vi "TIFF Add Image (array).vi"(8 "error in (no error)":errorcluster, 10 "IFD":refnum<class "IFD.lvclass">[](array[class]), 11 "TIFF in":refnum<class "TIFF.lvclass">) -> (0 "error out":errorcluster, 3 "TIFF out":refnum<class "TIFF.lvclass">)   [LabVIEW 2016, in "TIFF.lvclass"]
uses:
  TIFF.lvclass
  IFD/IFD.lvclass
  TIFF.lvclass/TIFF.ctl
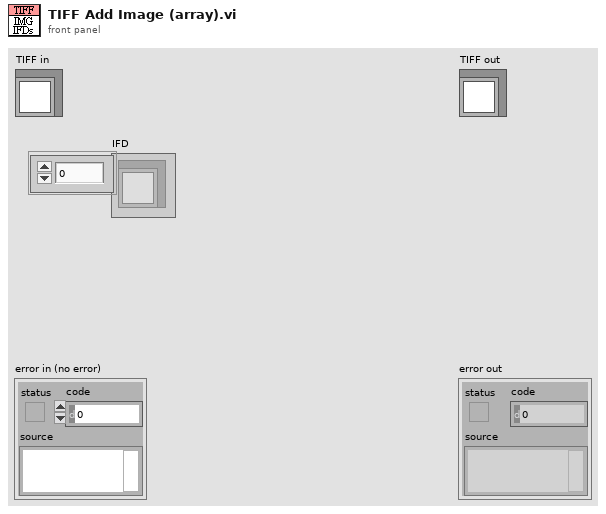
[diagram p1: front panel]
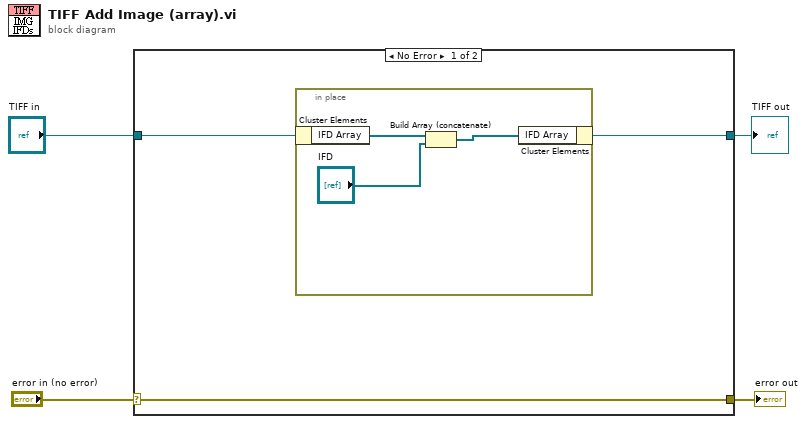
[diagram p0: block diagram]
diagram:
  n1 = case shown="No Error" "error in (no error)" {
    selector: "error in (no error)" -> [w7 w12]
    tunnel: [w7 w12] -> w3
    tunnel: [w5 w11] -> w1
    tunnel: "TIFF in" -> [w6 w11]
    frame No Error {
      n2 = in-place {
        n3 = in-place-cluster #1(w6) -> ("IFD Array"=w10:refnum<class "IFD.lvclass">[])
        n4 = Build Array (concatenate)(w10, "IFD") -> (w9:refnum<class "IFD.lvclass">[])
        n5 = in-place-cluster #1("IFD Array"=w9) -> (w5:refnum<class "TIFF.lvclass">)
      }
    }
    frame Error {
    }
  }
  "error out" <- w3
  "TIFF out" <- w1
